vi "Synaptic weights.vi"(1 "Activation functions, F":dbl[][](array[numeric]) format="%.3f", 2 "Feedbacks, C":dbl[][](array[numeric]) format="%.3f", 3 "Total error, e":dbl=1.0 min=-40.0 max=40.0 step=5.0 format="%.2f", 4 "Total control, u":dbl=1.0 min=-40.0 max=40.0 step=5.0 format="%.2f") -> (0 "Weights, W":dbl[][](array[numeric]) format="%.3f")   [LabVIEW 2022 SP3]
uses:
  <vilib>/Analysis/baseanly.llb/Real A x B.vi
  <vilib>/Analysis/Matrix/Numeric/Multiply/Multiply - R,RM.vi
  <vilib>/Analysis/NI_AALBase.lvlib
  <vilib>/Analysis/Matrix/NI_Matrix.lvlib
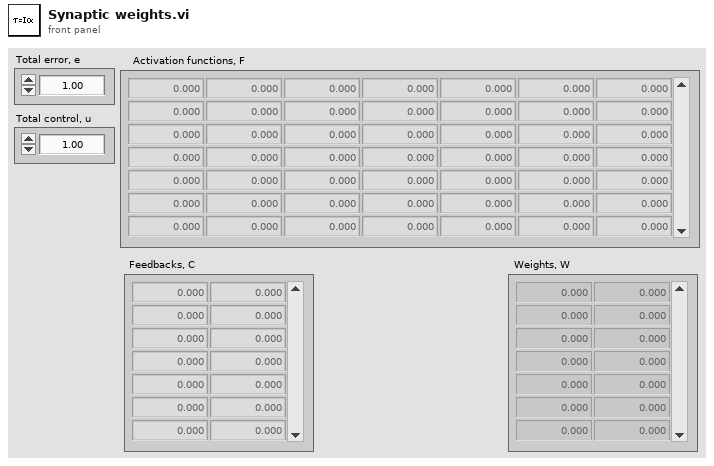
[diagram p1: front panel]
types:
  T1 = typedef "NI_Matrix.lvlib/RealMatrix.ctl" = dbl[][]
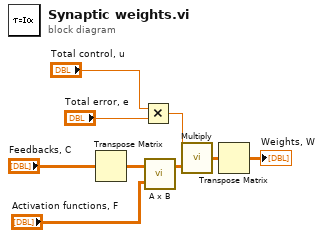
[diagram p0: block diagram]
diagram:
  n1 = Transpose Matrix(1:"Feedbacks, C") -> (0:w7:dbl[][])
  n2 = Multiply ("Multiply.vi")(x="Total control, u", y="Total error, e") -> (x*y=w2:dbl)
  n3 = call-poly <vilib>:"A x B.vi"("B"="Activation functions, F", "A"=w7) -> ("A x B"=w8:T1)  [unwired: 1 out]
  n4 = call-poly <vilib>:"Multiply.vi"("Real Matrix A"=w8, "Real Scalar c"=w2) -> ("c * A"=w5:T1)
  n5 = Transpose Matrix(1:w5) -> (0:→"Weights, W":T1)
